vi "Create or Write Workbook.vi"(8 "error in (no error)":errorcluster, 10 "File Name":path, 11 "IWorkbook Reference":refnum<k24>) -> (0 "error out":errorcluster, 3 "IWorkbook Reference Out":refnum<k24>)   [LabVIEW 2014]
uses:
  C:/PhaeronGit/LVNPOI/Resources/NPOI 2.1.1 dotnet2/NPOI.dll
  Resources/NPOI 2.1.1 dotnet2/NPOI.dll
  <vilib>/Utility/error.llb/Error Cluster From Error Code.vi
  <vilib>/ErrorRing/Error Ring.xnode
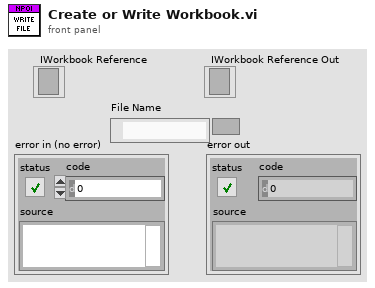
[diagram p1: front panel]
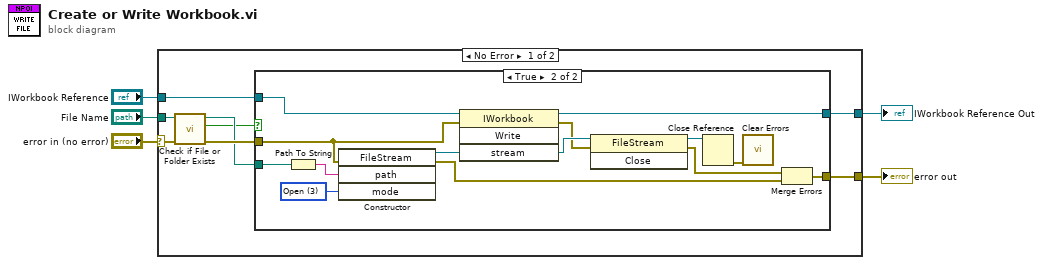
[diagram p0: block diagram]
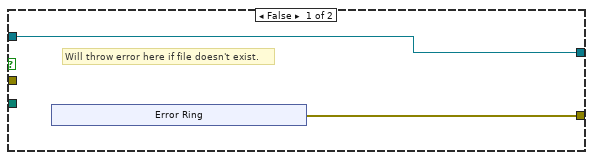
[diagram p2: hidden frame]
diagram:
  n1 = case shown="No Error" "error in (no error)" {
    selector: "error in (no error)" -> [w6 w34]
    tunnel: "IWorkbook Reference" -> [w13 w33]
    tunnel: [w12 w33] -> w4
    tunnel: [w11 w34] -> w3
    tunnel: "File Name" -> [w9 _]
    frame No Error {
      n2 = call <vilib>:"Check if File or Folder Exists.vi"("error in (no error)"=w6, "path"=w9) -> ("error out"=w10:errorcluster, "file or folder exists?"=w7:bool, "dup path"=w8:path)  [unwired: 7 in]
      n3 = case shown="True" w7 {
        tunnel: w13 -> [w14 w30]
        tunnel: [w14 w29] -> w12
        tunnel: [w15 w28] -> w11
        tunnel: w10 -> [_ w26]
        tunnel: w8 -> [_ w25]
        frame False {
          # "Will throw error here if file doesn't exist."
          n4 = xnode "Error Ring"() -> ("error out"=w15:errorcluster)
        }
        frame True {
          w31 = 3 items=["CreateNew"=1, "Create"=2, "Open"=3, "OpenOrCreate"=4, "Truncate"=5, "Append"=6] ("mode")
          n5 = Path To String(path=w25) -> (string=w32:string)
          n6 = constructor class="FileStream"(error in=w26, "path"=w32, "mode"=w31) -> (reference out=w23:refnum<k24>, error out=w27:errorcluster)  [unwired: 2 in, 3 out]
          n7 = invoke class="IWorkbook" method="Write"(reference=w30, error in=w26, "stream"=w23) -> (reference out=w29:refnum<k24>, error out=w21:errorcluster)  [unwired: 1 in, 2 out]
          n8 = invoke class="FileStream" method="Close"(reference=w23, error in=w21) -> (reference out=w22:refnum<k24>, error out=w20:errorcluster)  [unwired: 1 in, 1 out]
          n9 = Close Reference(reference=w22) -> (error out=w24:errorcluster)  [unwired: 1 in]
          n10 = call <vilib>:"Clear Errors.vi"("error in (no error)"=w24) -> ()  [unwired: 5 in, 2 out]
          n11 = Merge Errors(w20, w27) -> (w28:errorcluster)
        }
      }
    }
    frame Error {
    }
  }
  "IWorkbook Reference Out" <- w4
  "error out" <- w3
